vi "LV86_Morph_Thin.vi"(2 "Connectivity":enum16{"4", "6", "8"}(ring), 3 "Image in":T1 {"Dialogs" format="%.0b"}) -> (1 "Image out":T1 {"Dialogs" format="%.0b"})   [LabVIEW 2024]
doc: "Depending on the value of Connectivity, this VI can be used to remove single pixels isolated in the background and right angles along the edges of particles."
uses:
  <userlib>/ImageProcessing/QTLIB_2595_LV86/QT_Image.ctl
panel:
  # "Depending on the value of Connectivity, this \nVI can be used to remove single pixels isolated in the \nbackground and right angles along the edges of \nparticles."
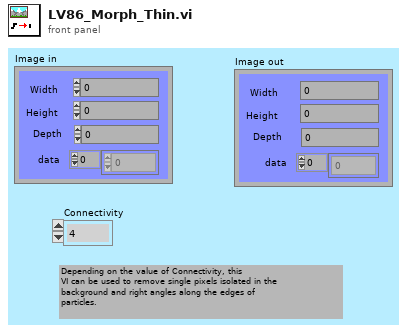
[diagram p1: front panel]
types:
  T1 = typedef "QT_Image.ctl" = cluster{"Width":i32, "Height":i32, "Depth":i32, "data":u8[], "Compressed data":u8[], "Color table":u32[], "Duration":i32, "Options":i32, "Timestamp":i32, "ID":i32, "Reserved":i32, "Dialogs":u32}
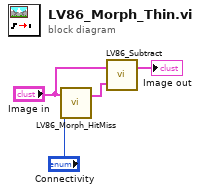
[diagram p0: block diagram]
diagram:
  n1 = call <userlib>:"LV86_Morph_HitMiss.vi"("Connectivity"="Connectivity", "Image in"="Image in") -> ("Image out"=w2:T1)  [unwired: 1 out]
  n2 = call <userlib>:"LV86_Subtract.vi"("Image 2"=w2, "Image"="Image in") -> ("Image Out"=→"Image out":T1)  [unwired: 1 in]
